vi "NIVS.FilterWaveforms.vi"(8 "error in (no error)":errorcluster, 11 "Cluster in":T1) -> (0 "error out":errorcluster, 3 "Cluster out":T1)   [LabVIEW 2015, in "Station.Execution.lvlib"]
uses:
  Station.Execution.lvlib
  Types/Main.StateVariables.ctl
  Types/Execute.UserEventRefs.ctl
  <vilib>/NI Veristand/Execution/Workspace/SystemStateRegEventRef.ctl
  <vilib>/NI Veristand/Execution/Workspace/Target State Info.ctl
  <vilib>/NI Veristand/Execution/Workspace/Target State.ctl
  <vilib>/NI Veristand/Execution/WaveformStreaming/Waveform Data Watcher Event Data (DBL).ctl
  <vilib>/NI Veristand/Execution/WaveformStreaming/WaveformStreamSpecification.ctl
  NationalInstruments.VeriStand.ClientAPI
  <vilib>/NI Veristand/Execution/Workspace/SystemStateEventRef.ctl
  <vilib>/NI Veristand/Execution/Workspace/WorkspaceAPI.ctl
  Types/UI.Tables.ctl
  Types/UI.Object.ctl
  Types/Waveforms.Info.ctl
  <vilib>/NI Veristand/Execution/WaveformStreaming/Registered Waveform Streams Data Event Refnum (DBL).ctl
  <vilib>/NI Veristand/Execution/WaveformStreaming/WaveformDataWatcherDBL.ctl
  <vilib>/NI Veristand/Execution/WaveformStreaming/WaveformStreamingAPI.ctl
  <vilib>/Utility/miscctls.llb/LVPositionTypeDef.ctl
  <vilib>/NI Veristand/Execution/Workspace/NI_VS Workspace ExecutionAPI.lvlib
  <vilib>/NI Veristand/Execution/WaveformStreaming/NI_VS Waveform Streaming Interface.lvlib
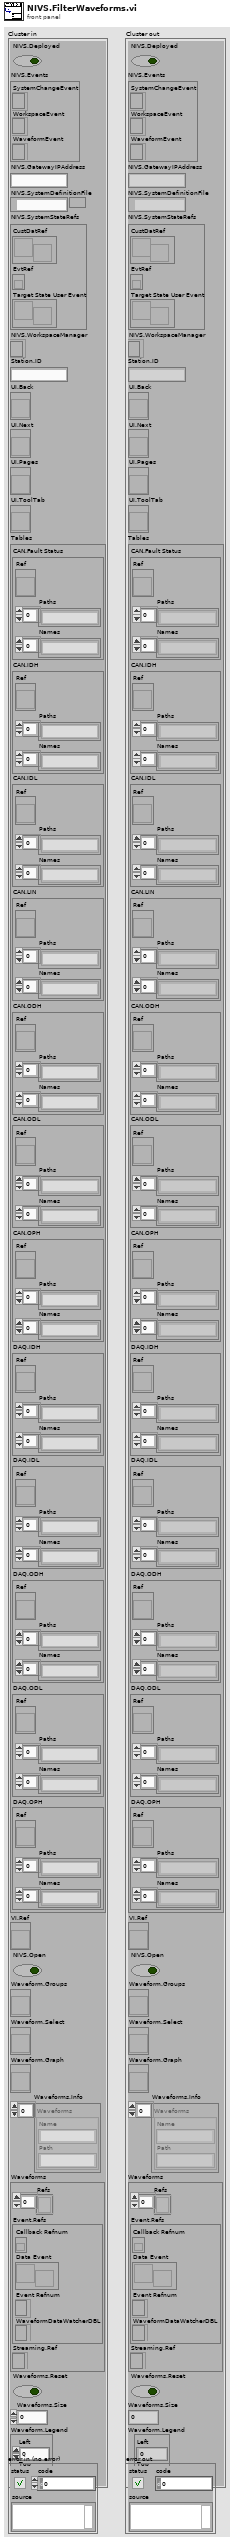
[diagram p1: front panel]
types:
  T1 = typedef "Station.Execution.lvlib/Main.StateVariables.ctl" = cluster{"NIVS.Deployed":bool, "NIVS.Events":T2, "NIVS.GatewayIPAddress":string, "NIVS.SystemDefinitionFile":path, "NIVS.SystemStateRefs":T4, "NIVS.WorkspaceManager":T5, "Station.ID":string, "UI.Back":refnum<vi>, "UI.Next":refnum<vi>, "UI.Pages":refnum<vi>, "UI.ToolTab":refnum<vi>, "Tables":T6, "VI.Ref":refnum<vi>, "NIVS.Open":bool, "Waveform.Groups":refnum<vi>, "Waveform.Select":refnum<vi>, "Waveform.Graph":refnum<vi>, "Waveforms.Info":T8[], "Waveforms":cluster{"Refs":T9[], "Event.Refs":T10, "Streaming.Ref":T12}, "Waveforms.Reset":bool, "Waveforms.Size":i32, "Waveform.Legend":T13}
  T2 = typedef "Station.Execution.lvlib/Execute.UserEventRefs.ctl" = cluster{"SystemChangeEvent":T3, "WorkspaceEvent":refnum<event-registration>, "WaveformEvent":refnum<event-registration>}
  T3 = typedef "NI_VS Workspace ExecutionAPI.lvlib/SystemStateRegEventRef.ctl" = refnum<event-registration>
  T4 = typedef "NI_VS Workspace ExecutionAPI.lvlib/SystemStateEventRef.ctl" = cluster{"CustDatRef":refnum<user-event>, "EvtRef":refnum<k27>, "Target State User Event":refnum<user-event>}
  T5 = typedef "NI_VS Workspace ExecutionAPI.lvlib/WorkspaceAPI.ctl" = refnum<k24>
  T6 = typedef "Station.Execution.lvlib/UI.Tables.ctl" = cluster{"CAN.Fault Status":T7, "CAN.IDH":T7, "CAN.IDL":T7, "CAN.LIN":T7, "CAN.ODH":T7, "CAN.ODL":T7, "CAN.OPH":T7, "DAQ.IDH":T7, "DAQ.IDL":T7, "DAQ.ODH":T7, "DAQ.ODL":T7, "DAQ.OPH":T7}
  T7 = typedef "Station.Execution.lvlib/UI.Object.ctl" = cluster{"Ref":refnum<vi>, "Paths":string[], "Names":string[]}
  T8 = typedef "Station.Execution.lvlib/Waveforms.Info.ctl" = cluster{"Name":string, "Path":string}
  T9 = typedef "NI_VS Waveform Streaming Interface.lvlib/WaveformStreamSpecification.ctl" = refnum<k24>
  T10 = typedef "NI_VS Waveform Streaming Interface.lvlib/Registered Waveform Streams Data Event Refnum (DBL).ctl" = cluster{"Callback Refnum":refnum<k27>, "Data Event":refnum<user-event>, "Event Refnum":refnum<event-registration>, "WaveformDataWatcherDBL":T11}
  T11 = typedef "NI_VS Waveform Streaming Interface.lvlib/WaveformDataWatcherDBL.ctl" = refnum<k24>
  T12 = typedef "NI_VS Waveform Streaming Interface.lvlib/WaveformStreamingAPI.ctl" = refnum<k24>
  T13 = typedef "LVPositionTypeDef.ctl" = cluster{"Left":i32, "Top":i32}
  T14 = typedef "NI_VS Workspace ExecutionAPI.lvlib/NodeInfo.ctl" = cluster{"Name":string, "FullPath":string, "Type":string, "IsChannel":bool, "Channel":cluster{"Unit":string, "Readable":bool, "Writable":bool, "Faultable":bool, "Scalable":bool, "RowDim":u32, "ColumnDim":u32, "Value Table Names":string[], "Value Table Values":dbl[]}, "IsWaveform":bool, "Waveform":cluster{"DataType":T15}}
  T15 = typedef "NI_VS Workspace ExecutionAPI.lvlib/Waveform Data Type.ctl" = enum16{"Double", "ComplexDouble"}
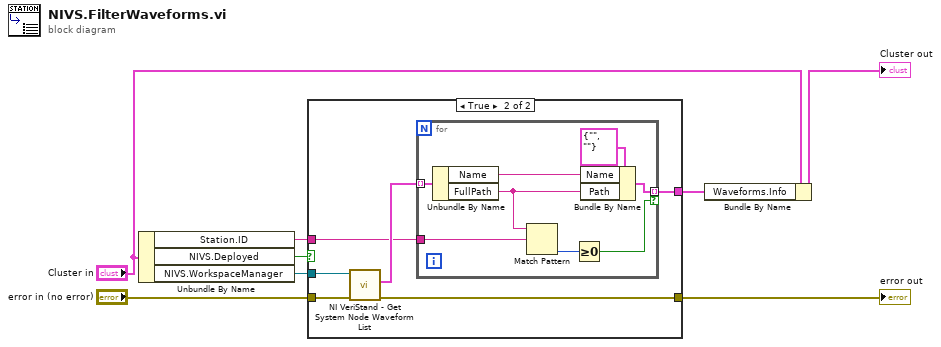
[diagram p0: block diagram]
diagram:
  n1 = Unbundle By Name("Cluster in") -> ("Station.ID"=w1:string, "NIVS.Deployed"=w8:bool, "NIVS.WorkspaceManager"=w2:T5)
  n2 = case shown="True" w8 {
    tunnel: w2 -> [_ w15]
    tunnel: "error in (no error)" -> [w9 w14]
    tunnel: [w9 w13] -> w4
    tunnel: [_ w11] -> w5
    tunnel: w1 -> [_ w10]
    frame False {
    }
    frame True {
      n3 = call <vilib>:"NI VeriStand - Get System Node Waveform List.vi"("error in (no error)"=w14, "WorkspaceManager in"=w15) -> ("error out"=w13:errorcluster, "Waveforms"=w12:T14[])  [unwired: 7 in, 1 out]
      n4 = for {
        tunnel: w12 -> [w23] mode=indexing
        tunnel: [w21] -> w11 mode=indexing if=w16
        tunnel: w10 -> [w18]
        n5 = Unbundle By Name(w23) -> ("Name"=w22:string, "FullPath"=w19:string)
        n6 = Match Pattern(string=w19, regular expression=w18) -> (offset past match=w17:i32)  [unwired: 1 in, 3 out]
        n7 = Greater Or Equal To 0?(x=w17) -> (x >= 0?=w16:bool)
        n8 = Bundle By Name(cluster=T8 {"Name"="", "Path"=""} ("Waveforms"), "Name"=w22, "Path"=w19) -> (w21:T8)
      }
    }
  }
  "error out" <- w4
  n9 = Bundle By Name(cluster="Cluster in", "Waveforms.Info"=w5) -> (→"Cluster out":T1)
